vi "GeometricPatternMatch_Setting_UI.vi"(0 "Vision_Image In":T3(plugin-control), 1 "Coord?":bool, 3 "Type":string, 5 "List ROI Ref":refnum<vi>, 7 "AlgIn":T2, 9 "ProjectName":string="CDF", 11 "error in (no error)":errorcluster, 12 "ParameterIn":string, 14 "RootPath":path) -> (6 "ParameerOut":string, 10 "IMAQ Curve Parameters.ctlCancel?":bool, 15 "error out":errorcluster)   [LabVIEW 2019]
uses:
  Controls/V_Analysis_Type.ctl
  <vilib>/vision/Pattern Matching.llb/IMAQ Match Range Setting.ctl
  Controls/_UI Command Cluster/Pattern Match_UI Command.ctl
  <vilib>/Utility/miscctls.llb/LVPointTypeDef.ctl
  Controls/Analysis_Setting.ctl
  Controls/Geometric Match/Analysis_Geometric PatternMatch_Parameter.ctl
  <vilib>/vision/Image Controls.llb/IMAQ Image.ctl
  11e1650d-9a27-4c98-b785-94bb4e51b252.vi
  fe4c8c9f-3b30-4d10-b5c7-71603a67618a.vi
  c6f29bbc-09ff-4359-9596-1a03bc10ebeb.vi
  7765c890-54c4-40a3-a063-9b2138e01ba1.vi
  ff688e6c-f413-41b3-9d93-3794729c7324.vi
  <vilib>/JDP Science/JSONtext/JSON text to Variant.vi
  <vilib>/JDP Science/JSONtext/Variant to JSON Text.vi
  <vilib>/vision/NI_Vision_Development_Module.lvlib
  <vilib>/userdefined/High Color/IMAQdx.ctl
panel:
  out "ListROI":T1
  out "Algout":T2=enum."G_PatternMatching"
  in  "SetROI":bool
  out "ROI":T1
  out "Template Image":T3(plugin-control)
  in  "Cancel":bool
  in  "Done":bool
  in  "PatternMatchTab":T4(tab)
  in  "Show Curve":bool
  in  "Curve Extraction":T5={"Extraction Mode"=0, "Edge Threshold"=75, "Edge Filter Size"=1, "Min Length"=25, "Row Search Step Size"=15, "Column Search Step Size"=15, "Max Endpoint Gap"=10, "Closed"=FALSE, "Subpixel"=FALSE} {"Edge Filter Size" items=["Fine", "Normal", "Contour Tracing"]; "Edge Threshold" min=0 max=255 step=1; "Extraction Mode" items=["Normal", "Uniform Regions"]}
  in  "Y Position Offset":i32
  in  "X Position Offset":i32
  in  "Match Parameters":T6={"Number of Matches Requested"=1, "Minimum Match Score"=750.0, "Angle Ranges"=[]} {"Angle Ranges"."End Angle" min=-360 max=360; "Angle Ranges"."Start Angle" min=-360 max=360; "Minimum Match Score" min=0 max=1000; "Number of Matches Requested" min=1 max=9999}
  in  "Match Mode":T7={"Rotation"=TRUE, "Scale"=FALSE, "Occlusion"=FALSE, "Reserved"=FALSE, "Reserved"=FALSE, "Reserved"=FALSE}
  in  "Range Settings":T8[](array[typedef])=[{"Match Constraints"=0, "Min"=-180.0, "Max"=180.0}] {"Match Constraints" items=["Rotation Angle (degrees)", "Scale Factor (%)", "Occlusion (%)"]}
  out "Matches (pixel)":T9(array[cluster]) {"Correlation Score" format="%.2f"; "Curve Score" format="%.2f"; "Curve Score" format="%.2f"; "Occlusion %" format="%.2f"; "Bounding Box"."y" format="%.2f"; "Bounding Box"."x" format="%.2f"; "Position"."y" format="%.2f"; "Position"."x" format="%.2f"; "Score" format="%.2f"; "Scale" format="%.2f"; "Angle" format="%.2f"}
  in  "Vision_Image":T3(plugin-control)
  in  "Run Algorithm":bool
  in  "SetTemplate":bool
  # "Range"
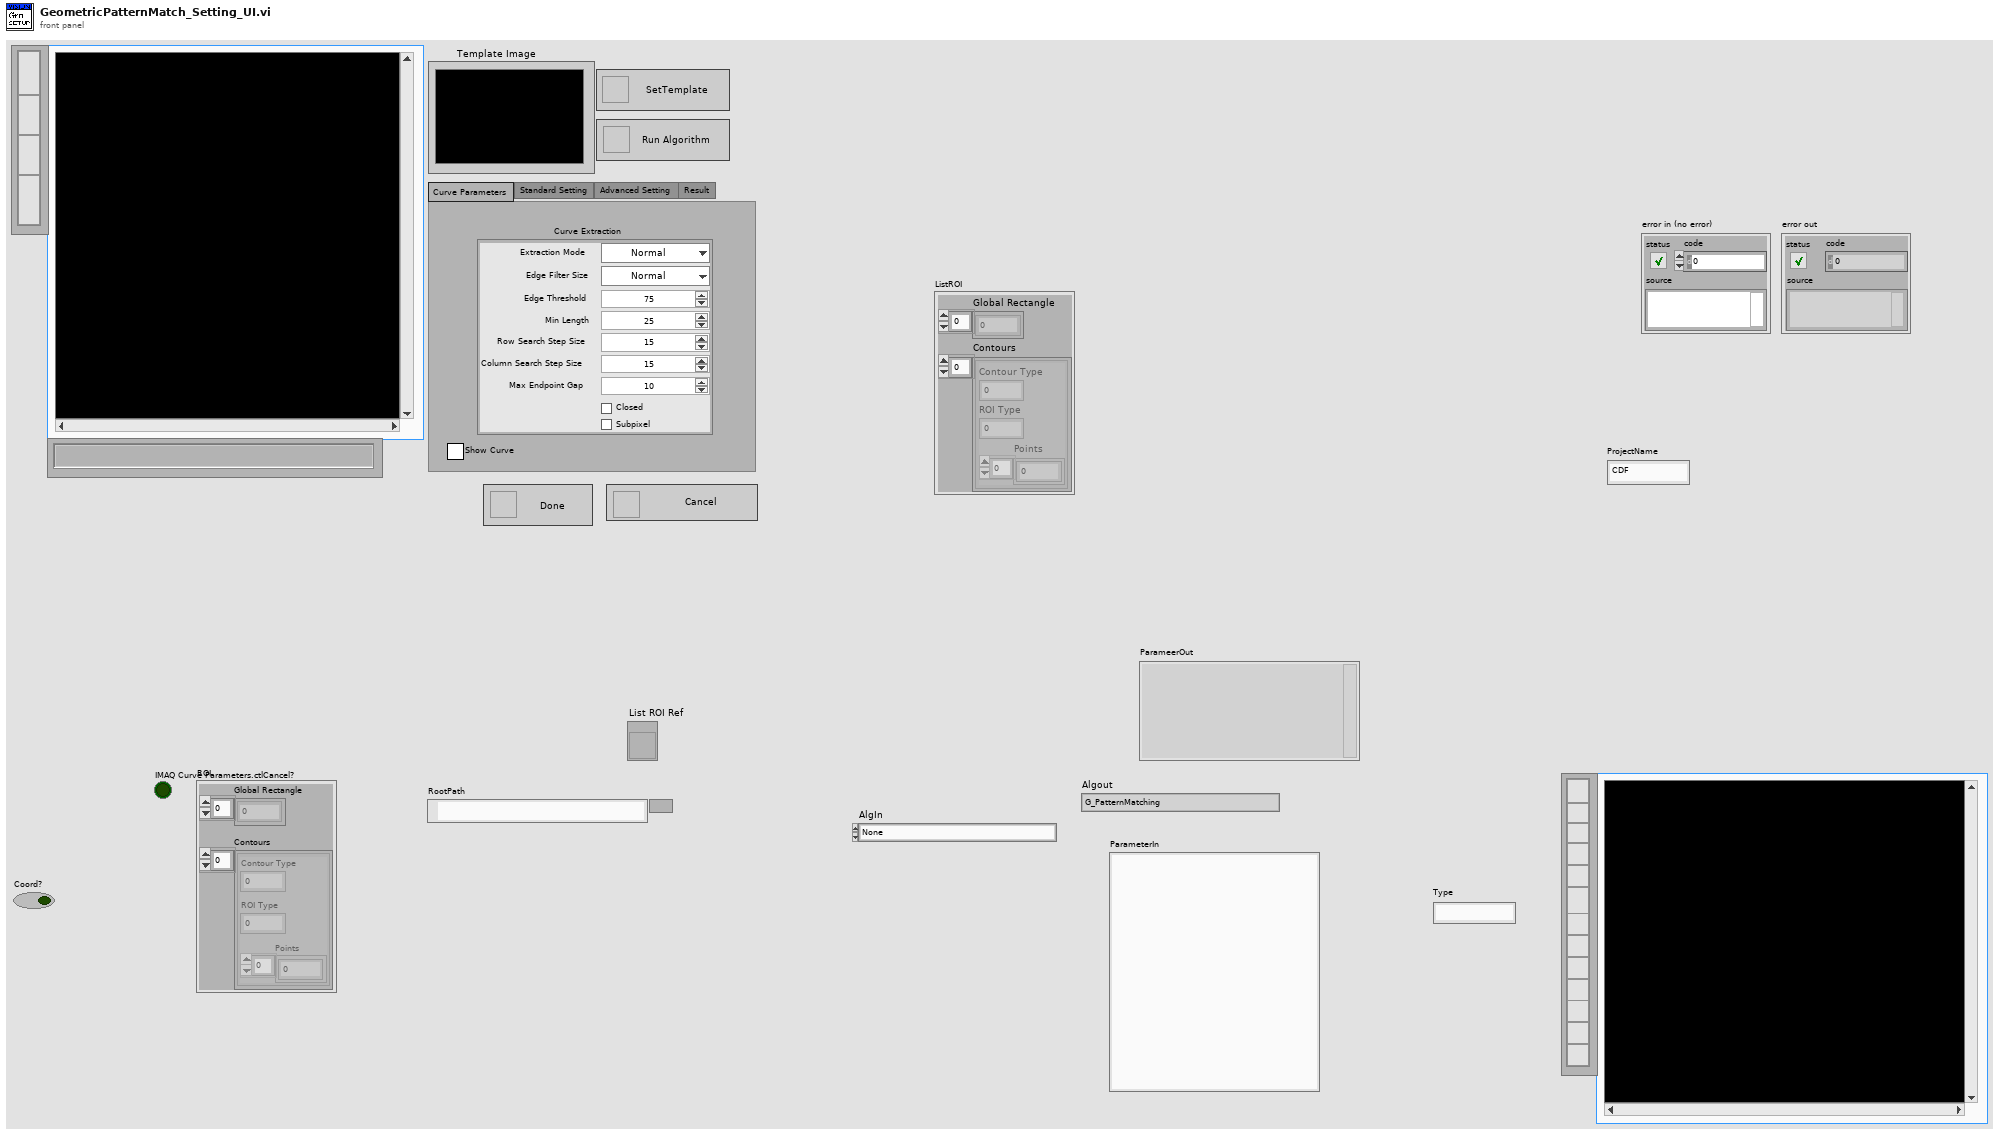
[diagram p1: front panel]
types:
  T1 = cluster{"Global Rectangle":i32[], "Contours":cluster{"Contour Type":u32, "ROI Type":u32, "Points":i32[]}[]}
  T2 = typedef "V_Analysis_Type.ctl" = enum16{"None", "C_Color Pattern Matching", "G_PatternMatching", "G_ShapeDectect", "G_GeometricMatch", "B_Area Check"}
  T3 = typedef "IMAQ Image.ctl" = refnum<image>
  T4 = enum32{"Curve Parameters", "Standard Setting", "Advanced Setting", "Result"}
  T5 = cluster{"Extraction Mode":u32, "Edge Threshold":i32, "Edge Filter Size":u32, "Min Length":i32, "Row Search Step Size":i32, "Column Search Step Size":i32, "Max Endpoint Gap":i32, "Closed":bool, "Subpixel":bool}
  T6 = cluster{"Number of Matches Requested":i32, "Minimum Match Score":sgl, "Angle Ranges":cluster{"Start Angle":sgl, "End Angle":sgl}[]}
  T7 = cluster{"Rotation":bool, "Scale":bool, "Occlusion":bool, "Reserved":bool, "Reserved":bool, "Reserved":bool}
  T8 = typedef "IMAQ Match Range Setting.ctl" = cluster{"Match Constraints":u32, "Min":dbl, "Max":dbl}
  T9 = cluster{"Position":cluster{"x":sgl, "y":sgl}, "Angle":sgl, "Scale":sgl, "Score":sgl, "Bounding Box":cluster{"x":sgl, "y":sgl}[], "Contrast Reversed":bool, "Occlusion %":sgl, "Curve Score":sgl, "Curve Score":sgl, "Correlation Score":sgl}[]
  T10 = typedef "Image Type" = u32
  T11 = typedef "Pattern Match_UI Command.ctl" = enum16{"Init", "Done", "Cancel", "RunAlgorithm", "SetTemplate", "SetROI", "ClearOverlay", "Load Template", "Draw Overlay", "Offset", "Draw Curve"}
  T12 = typedef "LVPointTypeDef.ctl" = cluster{"Horizontal":i16, "Vertical":i16}
  T13 = typedef "IMAQdx.ctl" = refnum<k21>
  T14 = typedef "Analysis_Geometric PatternMatch_Parameter.ctl" = cluster{"Curve Extraction":cluster{"Extraction Mode":u32, "Edge Threshold":i32, "Edge Filter Size":u32, "Min Length":i32, "Row Search Step Size":i32, "Column Search Step Size":i32, "Max Endpoint Gap":i32, "Closed":bool, "Subpixel":bool}, "X Position Offset":i32, "Y Position Offset":i32, "Match Parameters":cluster{"Number of Matches Requested":i32, "Minimum Match Score":sgl, "Angle Ranges":cluster{"Start Angle":sgl, "End Angle":sgl}[]}, "Template path":string, "Range Settings":T8[], "Match Mode":cluster{"Rotation":bool, "Scale":bool, "Occlusion":bool, "Reserved":bool, "Reserved":bool, "Reserved":bool}}
  T15 = typedef "Analysis_Setting.ctl" = cluster{"PreProcess":T2, "Parameter":string}
  T16 = enum8{"Enabled", "Disabled", "Disabled and Grayed Out"}
  T17 = typedef "ROI Descriptor" = cluster{"Global Rectangle":i32[], "Contours":cluster{"ID":enum32{"External", "Internal"}, "Type":u32, "Coordinates":i32[]}[]}
  T18 = cluster{"Position":cluster{"x":sgl, "y":sgl}, "Angle":sgl, "Scale":sgl, "Score":sgl, "Bounding Box":cluster{"x":sgl, "y":sgl}[]}[]
  T19 = typedef "IMAQ GM Match Report.ctl" = cluster{"Position":cluster{"x":sgl, "y":sgl}, "Angle":sgl, "Scale":sgl, "Score":sgl, "Bounding Box":cluster{"x":sgl, "y":sgl}[], "Contrast Reversed":bool, "Occlusion %":sgl, "Template Target Curve Score":sgl, "Target Template Curve Score":sgl, "Correlation Score":sgl}
  T20 = cluster{"Contour Type":u32, "ROI Type":u32, "Points":i32[]}[]
  T21 = cluster{"X Position Offset":i32, "Y Position Offset":i32}
  T22 = enum16{"Init", "Done", "Cancel", "RunAlgorithm", "SetTemplate", "SetROI", "ClearOverlay"}
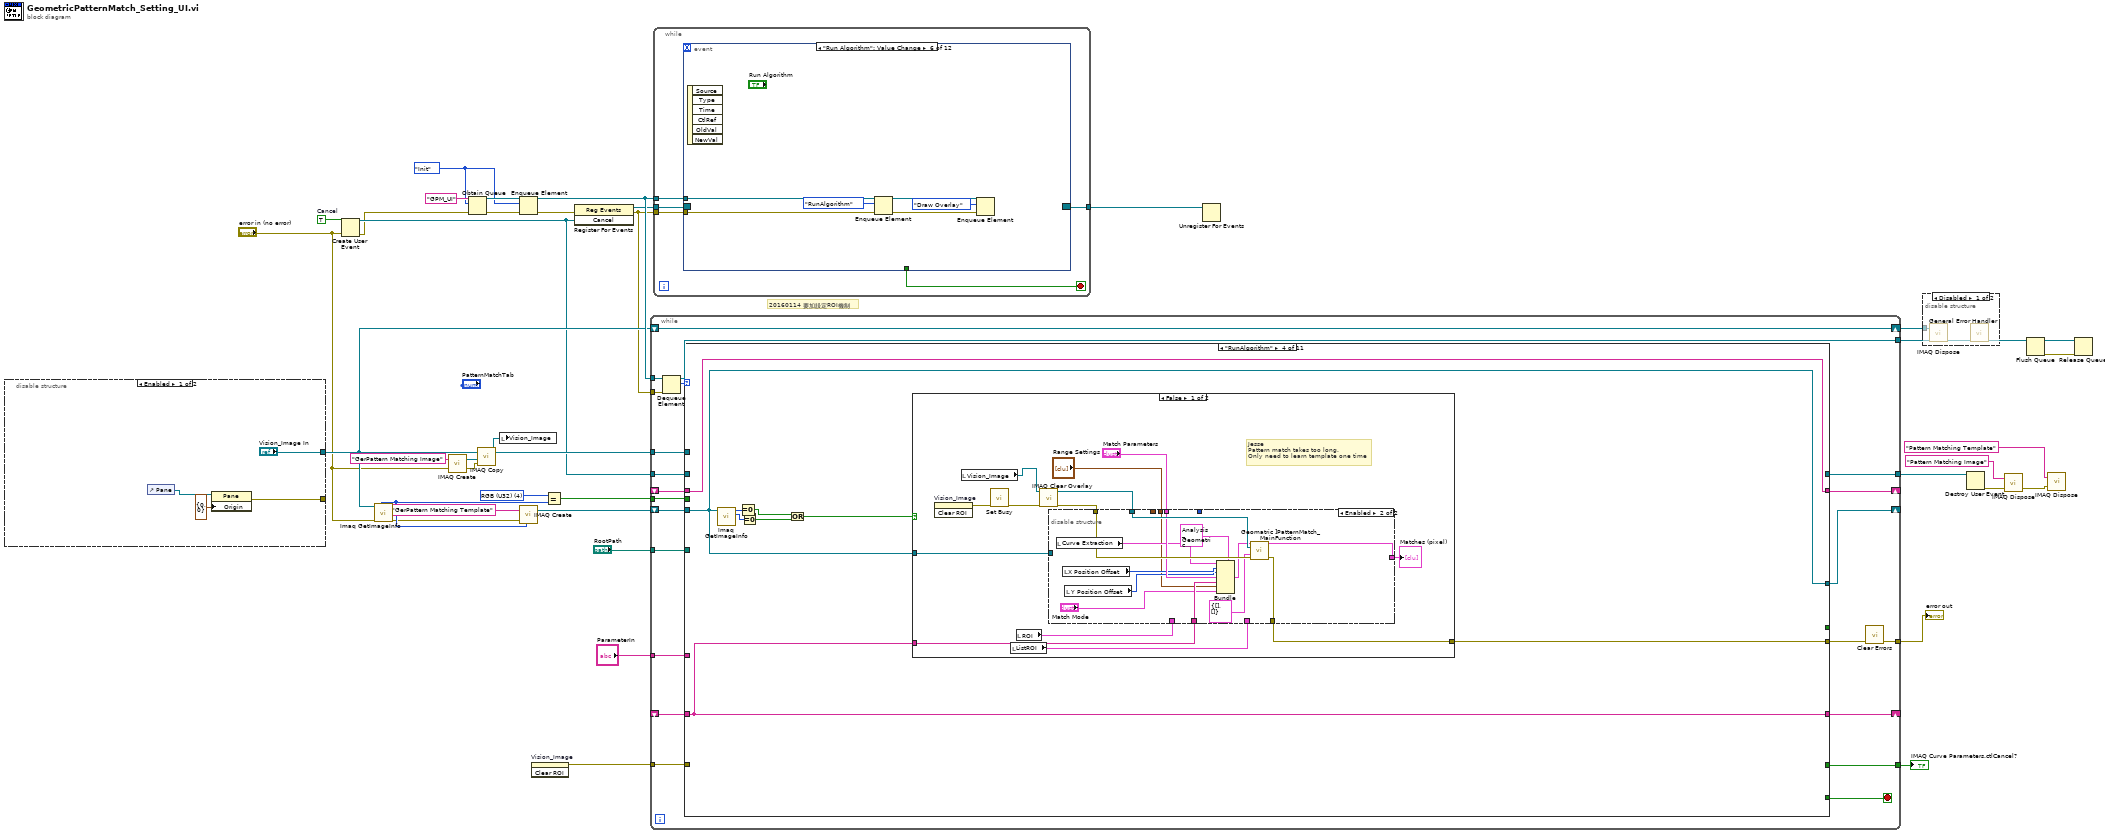
[diagram p0: block diagram]
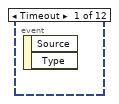
[diagram p2: hidden frame]
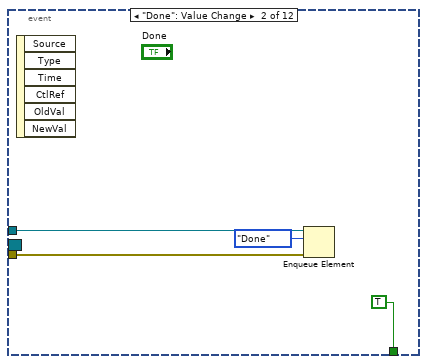
[diagram p3: hidden frame]
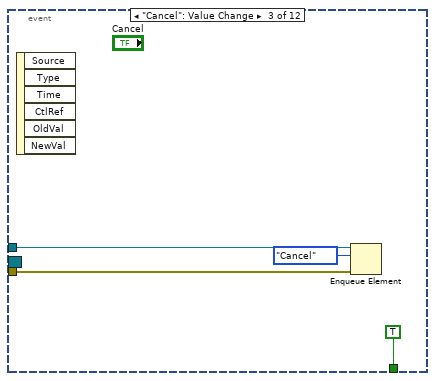
[diagram p4: hidden frame]
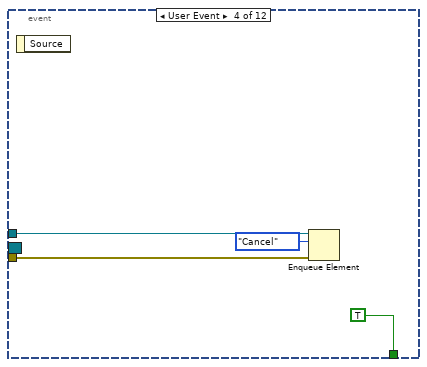
[diagram p5: hidden frame]
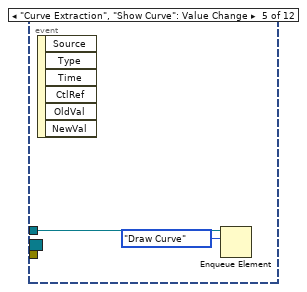
[diagram p6: hidden frame]
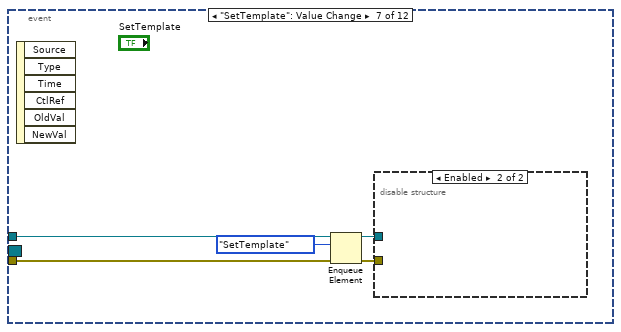
[diagram p7: hidden frame]
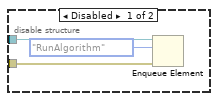
[diagram p8: hidden frame]
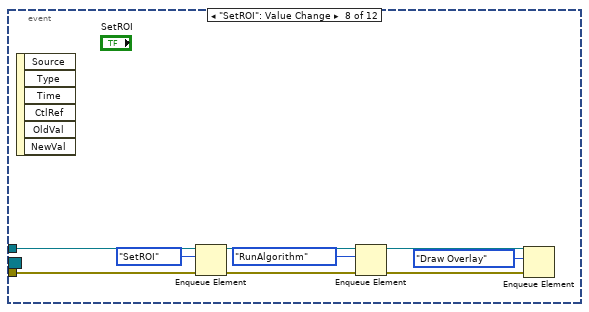
[diagram p9: hidden frame]
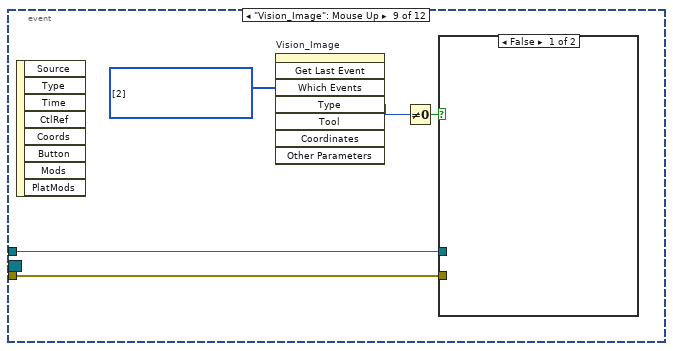
[diagram p10: hidden frame]
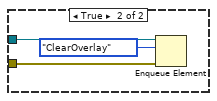
[diagram p11: hidden frame]
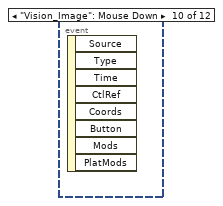
[diagram p12: hidden frame]
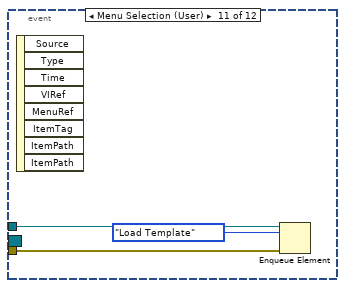
[diagram p13: hidden frame]
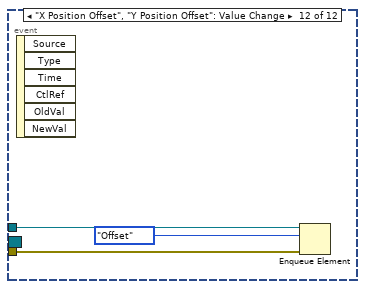
[diagram p14: hidden frame]
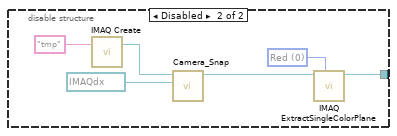
[diagram p15: hidden frame]
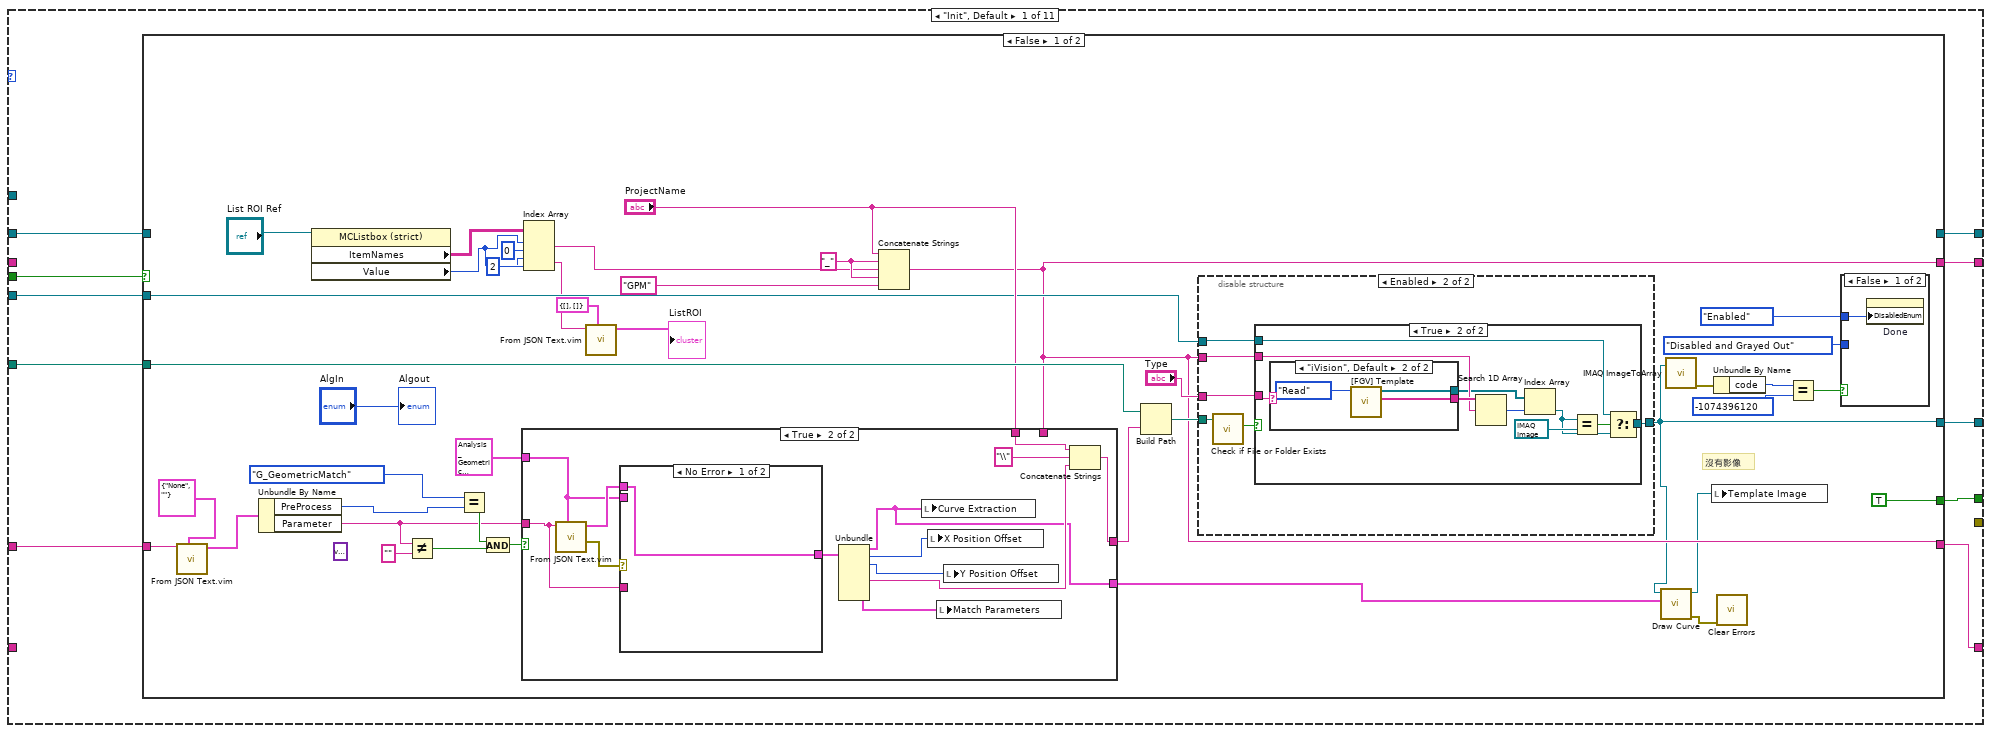
[diagram p17: hidden frame]
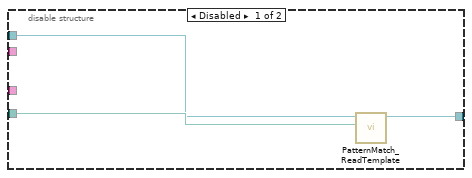
[diagram p18: hidden frame]
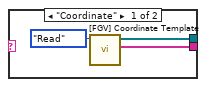
[diagram p20: hidden frame]
diagram:
  w18 = TRUE  # Cancel
  w20 = T10 4 items=["Grayscale (U8)", "Grayscale (I16)", "Grayscale (SGL)", "Complex (CSG)", "RGB (U32)", "HSL (U32)", "RGB (U64)", "Grayscale (U16)"] ("x")
  w19 = Pattern_Match_UI_Command."Init"
  # "20160114 要加設定ROI機制"
  n1 = disable-structure shown="Enabled" {
    disable-tunnel: ["Vision_Image In" w44] -> w24
    disable-tunnel: [w39 _] -> _
    frame Enabled {
      n2 = control-ref of="Pane"() -> (w41:refnum<vi>)
      n3 = property class="Pane"(reference=w41, "Origin"=T12 {"Horizontal"=0, "Vertical"=0}) -> (error out=w39:errorcluster)  [unwired: 1 in, 1 out]
    }
    frame Disabled {
      w43 = 0 items=["Red", "Green", "Blue", "Hue", "Saturation", "Luminance", "Value", "Intensity"] ("Color Plane")
      n4 = call "IMAQ Create"("Image Name"="tmp") -> ("New Image"=w46:T3)  [unwired: 4 in, 1 out]
      n5 = call "Camera_Snap.vi"("Camera Session In"=T13 "cam0", "Image In"=w46) -> ("New Image"=w45:T3)  [unwired: 8 in, 1 out]
      n6 = call "IMAQ ExtractSingleColorPlane"("Color Plane"=w43, "Image Src"=w45) -> ("Image Dst Out"=w44:T3)  [unwired: 2 in, 7 out]
    }
  }
  n7 = Create User Event(user event datatype=w18, error in="error in (no error)") -> (user event=w15:refnum<user-event>, error out=w6:errorcluster)
  n8 = call "Imaq GetImageInfo"("error in (no error)"="error in (no error)", "Image"=w24) -> ("error out"=w4:errorcluster, "Image Type"=w21:T10)  [unwired: 2 in, 6 out]
  n9 = call "IMAQ Create"("Image Name"="GerPattern Matching Image", "error in (no error)"="error in (no error)") -> ("New Image"=w33:T3, "error out"=w5:errorcluster)  [unwired: 3 in]
  n10 = Obtain Queue(name (unnamed)="GPM_UI", element data type=w19, error in (no error)=w6) -> (queue out=w30:refnum<queue>, error out=w29:errorcluster)  [unwired: 2 in, 1 out]
  n11 = call "IMAQ Copy"("error in (no error)"=w5, "Image Dst"=w33, "Image Src"=w24) -> ("Image Dst Out"=w32:T3)  [unwired: 3 in, 1 out]
  n12 = local write "Vision_Image"(w32) -> ()
  n13 = Enqueue Element(queue=w30, element=w19, error in (no error)=w29) -> (queue out=w26:refnum<queue>, error out=w12:errorcluster)  [unwired: 1 in, 1 out]
  n14 = call "IMAQ Create"("Image Name"="GerPattern Matching Template", "Image Type"=w21, "error in (no error)"=w4) -> ("New Image"=w23:T3)  [unwired: 2 in, 1 out]
  n15 = invoke on="Vision_Image" class="ImageControl" method="Clear ROI"() -> (error out=w35:errorcluster)  [unwired: 3 in, 2 out]
  n16 = Equal?(x=w20, y=w21) -> (x = y?=w16:bool)
  n17 = register-events(error in=w12, w15) -> (reference out=w17:refnum<event-registration>, error out=w11:errorcluster)  [unwired: 1 in]
  n18 = while {
    shift-right: [w70] -> w38
    shift-left: w24 -> [w70]
    tunnel: [w66] -> w37
    tunnel: w35 -> [w52]
    tunnel: w32 -> [w69]
    tunnel: w26 -> [w64]
    tunnel: w11 -> [w62]
    tunnel: [w61] -> w25
    shift-right: [w60] -> _
    shift-left: _ -> [w59]
    shift-right: [w57] -> _
    shift-left: w23 -> [w68]
    shift-right: [w58] -> _
    shift-left: _ -> [w67]
    tunnel: "RootPath" -> [w56]
    tunnel: w16 -> [w55]
    tunnel: w15 -> [w54]
    tunnel: [w53] -> w14
    tunnel: [w51] -> w2
    tunnel: "ParameterIn" -> [w49]
    stop <- w65 stop-if-true
    n19 = Dequeue Element(queue=w64, error in (no error)=w62) -> (queue out=w61:refnum<queue>, element=w63:T11)  [unwired: 1 in, 2 out]
    n20 = case shown="\"RunAlgorithm\"" w63 {
      tunnel: [_ TRUE w205 _ _ _ _ _ _ _ _] -> w65
      tunnel: w69 -> [_ w194 w204 _ w262 _ _ _ _ _ w447]
      tunnel: w68 -> [w75 _ w203 w209 w264 w311 w380 w390 w404 w419 w445]
      tunnel: [_ _ w205 _ _ _ _ _ _ _ _] -> w66
      tunnel: w67 -> [_ w183 w201 w207 w263 w312 w381 w391 w405 w424 w444]
      tunnel: [w79 w193 w202 w214 w265 w313 w382 w392 w406 _ w446] -> w60
      tunnel: w59 -> [_ w193 w202 w214 w265 w313 w382 w392 w406 _ w446]
      tunnel: [w77 w183 w201 w207 w263 w312 w381 w391 w405 w424 w444] -> w58
      tunnel: [w80 T3 refnum ("Template Out") T3 refnum ("Template Out") w209 w264 w308 w380 w390 w396 w426 w445] -> w57
      tunnel: [w78 FALSE _ _ _ w310 _ _ _ _ _] -> _
      tunnel: w56 -> [w76 _ _ _ _ w309 _ _ w403 w425 _]
      tunnel: w55 -> [w74 _ _ _ _ _ _ _ _ _ _]
      tunnel: w54 -> [w73 w190 w199 _ _ _ _ _ _ _ _]
      tunnel: [w72 w190 w199 _ _ _ _ _ _ _ _] -> w53
      tunnel: w52 -> [_ _ _ _ w259 _ _ _ _ _ _]
      tunnel: [_ _ _ w206 _ _ _ _ _ _ _] -> w50
      tunnel: w49 -> [w71 _ _ _ _ _ _ _ _ _ _]
      frame "Init", Default {
        n21 = case shown="False" w74 {
          tunnel: [w83 _] -> w80
          tunnel: [w87 _] -> w79
          tunnel: [TRUE _] -> w78
          tunnel: [w87 _] -> w77
          tunnel: w76 -> [w120 _]
          tunnel: w75 -> [w110 _]
          tunnel: w73 -> [_ w176]
          tunnel: [_ w174] -> w72
          tunnel: w71 -> [w89 _]
          frame False {
            (unwired) variant
            w117 = "_" ("string")
            # "沒有影像"
            n22 = call "From JSON Text.vim"("Data Type and Default Value"=T15 {"PreProcess"=enum."None", "Parameter"=""} ("Analysis_Setting In"), "JSON"=w89) -> ("Data out"=w90:T15)  [unwired: 8 in, 1 out]
            n23 = Unbundle By Name(w90) -> ("PreProcess"=w88:T2, "Parameter"=w112:string)
            n24 = property class="MCListbox (strict)"(reference="List ROI Ref") -> ("ItemNames"=w97:string[][], "Value"=w96:i32)  [unwired: 1 in, 2 out]
            n25 = Not Equal?(x=w112, y="") -> (x != y?=w115:bool)
            n26 = Equal?(x=V_Analysis_Type."G_GeometricMatch", y=w88) -> (x = y?=w116:bool)
            n27 = And(x=w116, y=w115) -> (x .and. y?=w113:bool)
            n28 = Index Array(array=w97, index (row) #1=w96, index (col) #1=0 ("disabled index (col)"), index (row) #2=w96, index (col) #2=2 ("disabled index (col)")) -> (element #1=w95:string, element #2=w93:string)
            n29 = call "From JSON Text.vim"("Data Type and Default Value"=T1 {"Global Rectangle"=[], "Contours"=[]} ("ROI"), "JSON"=w93) -> ("Data out"=→"ListROI":T1)  [unwired: 8 in, 1 out]
            n30 = Concatenate Strings("ProjectName", w117, w95, w117, "GPM" ("string")) -> (w87:string)
            n31 = case shown="True" w113 {
              tunnel: [w152 w166] -> w86
              tunnel: "ProjectName" -> [w153 w168]
              tunnel: w112 -> [_ w170]
              tunnel: w87 -> [w154 _]
              tunnel: T14 {"Curve Extraction"={"Extraction Mode"=0, "Edge Threshold"=75, "Edge Filter Size"=1, "Min Length"=25, "Row Search Step Size"=15, "Column Search Step Size"=15, "Max Endpoint Gap"=10, "Closed"=FALSE, "Subpixel"=FALSE}, "X Position Offset"=0, "Y Position Offset"=0, "Match Parameters"={"Number of Matches Requested"=1, "Minimum Match Score"=750.0, "Angle Ranges"=[]}, "Template path"="", "Range Settings"=[], "Match Mode"={"Rotation"=TRUE, "Scale"=FALSE, "Occlusion"=FALSE, "Reserved"=FALSE, "Reserved"=FALSE, "Reserved"=FALSE}} ("Cluster") -> [w151 w165]
              tunnel: [w150 w159] -> w82
              frame False {
                n32 = invoke on="Y Position Offset" class="DigNum (strict)" method="Reinit To Default"() -> ()  [unwired: 3 in, 3 out]
                n33 = invoke on="X Position Offset" class="DigNum (strict)" method="Reinit To Default"() -> ()  [unwired: 3 in, 3 out]
                n34 = Unbundle By Name(w151) -> ("Curve Extraction"=w150:T5)
                n35 = case shown="True" "Coord?" {
                  frame False {
                    n36 = invoke on="Match Parameters" class="Clust (strict)" method="Reinit To Default"() -> ()  [unwired: 3 in, 3 out]
                  }
                  frame True {
                    n37 = local write "Match Parameters"(T6 {"Number of Matches Requested"=1, "Minimum Match Score"=750.0, "Angle Ranges"=[{"Start Angle"=0.0, "End Angle"=360.0}]} ("Match Parameters")) -> ()
                  }
                }
                n38 = Concatenate Strings(w153, "\\" ("string"), w154) -> (w152:string)
                "ROI" <- T1 {"Global Rectangle"=[], "Contours"=[]} ("ROI")
              }
              frame True {
                n39 = call "From JSON Text.vim"("Data Type and Default Value"=w165, "JSON"=w170) -> ("error out"=w171:errorcluster, "Data out"=w169:T14)  [unwired: 8 in]
                n40 = case shown="No Error" w171 {
                  tunnel: w170 -> [_ _]
                  tunnel: [w172 w173] -> w164
                  tunnel: w169 -> [w172 _]
                  tunnel: w165 -> [_ w173]
                  frame No Error {
                  }
                  frame Error {
                  }
                }
                n41 = Unbundle(w164) -> ("Curve Extraction"=w159:T5, "X Position Offset"=w163:i32, "Y Position Offset"=w162:i32, "Match Parameters"=w161:T6, "Template path"=w160:string)  [unwired: 2 out]
                n42 = local write "Curve Extraction"(w159) -> ()
                n43 = local write "X Position Offset"(w163) -> ()
                n44 = local write "Match Parameters"(w161) -> ()
                n45 = local write "Y Position Offset"(w162) -> ()
                n46 = Concatenate Strings(w168, "\\" ("string"), w160) -> (w166:string)
              }
            }
            n47 = Build Path(base path=w120, name or relative path=w86) -> (appended path=w111:path)
            n48 = disable-structure shown="Enabled" {
              disable-tunnel: w111 -> [w124 w129]
              disable-tunnel: w110 -> [w123 w126]
              disable-tunnel: [w122 w127] -> w83
              disable-tunnel: w87 -> [_ w130]
              disable-tunnel: "Type" -> [_ w125]
              frame Disabled {
                n49 = call "PatternMatch_ReadTemplate.vi"("template path"=w124, "Template"=w123) -> ("Template Out"=w122:T3)  [unwired: 8 in, 1 out]
              }
              frame Enabled {
                n50 = call <vilib>:"Check if File or Folder Exists.vi"("path"=w129) -> ("file or folder exists?"=w128:bool)  [unwired: 8 in, 2 out]
                n51 = case shown="True" w128 {
                  tunnel: w130 -> [_ w140]
                  tunnel: [w131 w132] -> w127
                  tunnel: w126 -> [w131 w134]
                  tunnel: w125 -> [_ w137]
                  frame False {
                  }
                  frame True {
                    n52 = case shown="\"iVision\", Default" w137 {
                      tunnel: [w143 w146] -> w141
                      tunnel: [w144 w145] -> w138
                      frame "Coordinate" {
                        n53 = call "[FGV] Coordinate Template.vi"("Command"=enum16{"Initialize", "Save", "Read"}."Read") -> ("Image Name Array"=w143:string[], "Image Array"=w144:T3[])  [unwired: 8 in, 1 out]
                      }
                      frame "iVision", Default {
                        n54 = call "[FGV] Template.vi"("Command"=enum16{"Initialize", "Save", "Read"}."Read") -> ("Image Name Array"=w146:string[], "Image Array"=w145:T3[])  [unwired: 8 in, 1 out]
                      }
                    }
                    n55 = Search 1D Array(1D array=w141, element=w140) -> (index of element=w139:i32)  [unwired: 1 in]
                    n56 = Index Array(array=w138, index=w139) -> (element=w133:T3)
                    n57 = Equal?(x=w133, y=T3 refnum) -> (x = y?=w135:bool)
                    n58 = Select(t=w134, s=w135, f=w133) -> (s? t:f=w132:T3)
                  }
                }
              }
            }
            n59 = call "Draw Curve.vi"("Curve Extraction"=w82, "Refnum in"=w83) -> ("error out"=w81:errorcluster, "Refnum out"=w84:T3)  [unwired: 8 in]
            n60 = call "IMAQ ImageToArray"("Image"=w83) -> ("error out"=w107:errorcluster)  [unwired: 3 in, 4 out]
            n61 = local write "Template Image"(w84) -> ()
            n62 = Unbundle By Name(w107) -> ("code"=w106:i32)
            n63 = call <vilib>:"Clear Errors.vi"("error in (no error)"=w81) -> ()  [unwired: 5 in, 2 out]
            n64 = Equal?(x=w106, y=-1074396120) -> (x = y?=w104:bool)
            n65 = case shown="False" w104 {
              tunnel: T16."Disabled and Grayed Out" ("Disabled") -> [_ w149]
              tunnel: T16."Enabled" ("Disabled") -> [w148 _]
              frame False {
                n66 = property on="Done" class="Bool"("DisabledEnum"=w148) -> ()  [unwired: 2 in, 2 out]
              }
              frame True {
                n67 = property on="Done" class="Bool"("DisabledEnum"=w149) -> ()  [unwired: 2 in, 2 out]
              }
            }
            "Algout" <- "AlgIn"
          }
          frame True {
            # "輸入進來若是RGB則關閉"
            n68 = One Button Dialog(message="The Input Image Error,Image RGB", button name ("OK")="Cancel") -> (true=w175:bool)
            n69 = Generate User Event(user event=w176, event data cluster=w175) -> (user event out=w174:refnum<user-event>)  [unwired: 2 in, 1 out]
          }
        }
      }
      frame "Done" {
        w196 = T15 {"PreProcess"=enum."None", "Parameter"=""}  # Analysis_Setting
        n70 = call "IMAQ Dispose"("Image"=w194) -> ()  [unwired: 5 in, 1 out]
        n71 = local read "Y Position Offset"() -> (w181:i32)
        n72 = local read "X Position Offset"() -> (w182:i32)
        n73 = local read "Curve Extraction"() -> (w184:T5)
        n74 = local read "Match Parameters"() -> (w195:T6)
        n75 = local read "Range Settings"() -> (w180:T8[])
        n76 = local read "Match Mode"() -> (w179:T7)
        n77 = Bundle By Name(cluster=T14 {"Curve Extraction"={"Extraction Mode"=0, "Edge Threshold"=75, "Edge Filter Size"=1, "Min Length"=25, "Row Search Step Size"=15, "Column Search Step Size"=15, "Max Endpoint Gap"=10, "Closed"=FALSE, "Subpixel"=FALSE}, "X Position Offset"=0, "Y Position Offset"=0, "Match Parameters"={"Number of Matches Requested"=1, "Minimum Match Score"=750.0, "Angle Ranges"=[]}, "Template path"="", "Range Settings"=[], "Match Mode"={"Rotation"=TRUE, "Scale"=FALSE, "Occlusion"=FALSE, "Reserved"=FALSE, "Reserved"=FALSE, "Reserved"=FALSE}} ("Cluster"), "Curve Extraction"=w184, "Match Parameters"=w195, "X Position Offset"=w182, "Y Position Offset"=w181, "Template path"=w183, "Range Settings"=w180, "Match Mode"=w179) -> (w189:T14)
        n78 = call "To JSON Text.vim"("Anything"=w189) -> ("<JSON>"=w188:string)  [unwired: 9 in, 1 out]
        n79 = Bundle By Name(cluster=w196, "PreProcess"=V_Analysis_Type."G_GeometricMatch" ("Analysis"), "Parameter"=w188) -> (w187:T15)
        n80 = call "To JSON Text.vim"("Anything"=w187) -> ("<JSON>"=→"ParameerOut":string)  [unwired: 9 in, 1 out]
      }
      frame "Cancel" {
        w205 = TRUE
        n81 = call "IMAQ Dispose"("Image"=w203) -> ()  [unwired: 5 in, 1 out]
        n82 = call "IMAQ Dispose"("Image"=w204) -> ()  [unwired: 5 in, 1 out]
      }
      frame "RunAlgorithm" {
        n83 = call "Imaq GetImageInfo"("Image"=w209) -> ("Y Resolution"=w213:i32, "X Resolution"=w212:i32)  [unwired: 3 in, 6 out]
        n84 = Equal To 0?(x=w212) -> (x = 0?=w211:bool)
        n85 = Equal To 0?(x=w213) -> (x = 0?=w210:bool)
        n86 = Or(x=w211, y=w210) -> (x .or. y?=w208:bool)
        n87 = case shown="False" w208 {
          tunnel: w209 -> [w221 _]
          tunnel: w207 -> [w220 _]
          tunnel: [w219 _] -> w206
          frame False {
            # "Jesse\nPattern match takes too long.\nOnly need to learn template one time"
            n88 = invoke on="Vision_Image" class="ImageControl" method="Clear ROI"() -> (error out=w227:errorcluster)  [unwired: 3 in, 2 out]
            n89 = local read "Vision_Image"() -> (w215:T3)
            n90 = call <vilib>:"Set Busy.vi"("error in (no error)"=w227) -> ("error out"=w226:errorcluster)  [unwired: 9 in, 1 out]
            n91 = local read "ListROI"() -> (w218:T1)
            n92 = local read "ROI"() -> (w222:T1)
            n93 = call "IMAQ Clear Overlay"("error in (no error)"=w226, "Image"=w215) -> ("error out"=w223:errorcluster, "Image Out"=w225:T3)  [unwired: 8 in]
            n94 = disable-structure shown="Enabled" {
              disable-tunnel: w221 -> [w237 _]
              disable-tunnel: w223 -> [w236 w251]
              disable-tunnel: "Match Parameters" -> [w234 w247]
              disable-tunnel: _ -> [w233 _]
              disable-tunnel: _ -> [w232 _]
              disable-tunnel: w225 -> [w231 w252]
              disable-tunnel: [w230 w253] -> w217
              disable-tunnel: w222 -> [w228 _]
              disable-tunnel: w220 -> [_ w250]
              disable-tunnel: [_ w249] -> w219
              disable-tunnel: w218 -> [_ _]
              disable-tunnel: "Range Settings" -> [_ w242]
              frame Disabled {
                w239 = 0 items=["All", "Low Discrepancy Sampling", "Grayscale Value Pyramid", "Gradients Pyramid"] ("Algorithm")
                n95 = call "IMAQ Learn Pattern 4"("Algorithm"=w239, "error in (no error)"=w236, "Angle Range"=cluster{"Start Angle":sgl, "End Angle":sgl} {"Start Angle"=0.0, "End Angle"=360.0}, "Image"=w237) -> ("error out"=w235:errorcluster, "Template Image Out"=w229:T3)  [unwired: 5 in, 1 out]
                n96 = call "IMAQ Match Pattern 4"("Image"=w231, "Algorithm"=w233, "Template Image"=w229, "ROI Descriptor"=w228, "Parameters"=w234, "error in (no error)"=w235, "Advanced Options"=w232) -> ("Matches (pixel)"=w230:T18)  [unwired: 4 in, 4 out]
              }
              frame Enabled {
                n97 = local read "Curve Extraction"() -> (w246:T5)
                n98 = local read "X Position Offset"() -> (w245:i32)
                n99 = local read "Y Position Offset"() -> (w244:i32)
                n100 = Bundle(cluster=T14 {"Curve Extraction"={"Extraction Mode"=0, "Edge Threshold"=75, "Edge Filter Size"=1, "Min Length"=25, "Row Search Step Size"=15, "Column Search Step Size"=15, "Max Endpoint Gap"=10, "Closed"=FALSE, "Subpixel"=FALSE}, "X Position Offset"=0, "Y Position Offset"=0, "Match Parameters"={"Number of Matches Requested"=1, "Minimum Match Score"=750.0, "Angle Ranges"=[]}, "Template path"="", "Range Settings"=[], "Match Mode"={"Rotation"=TRUE, "Scale"=FALSE, "Occlusion"=FALSE, "Reserved"=FALSE, "Reserved"=FALSE, "Reserved"=FALSE}} ("Cluster"), "Curve Extraction"=w246, "X Position Offset"=w245, "Y Position Offset"=w244, "Match Parameters"=w247, "Template path"=w250, "Range Settings"=w242, "Match Mode"="Match Mode") -> (w243:T14)
                n101 = call "Geomatric ]PatternMatch_MainFunction.vi"("Geomatric Match Parameter"=w243, "Vision_Image In"=w252, "ROI Descriptor"=T17 {"Global Rectangle"=[], "Contours"=[]}, "error in"=w251) -> ("Matches (pixel)"=w253:T19[], "error out"=w249:errorcluster)  [unwired: 7 in, 3 out]
              }
            }
            "Matches (pixel)" <- w217
          }
          frame True {
            n102 = One Button Dialog(message="No Template is Set~!!!\nPlease Set Template Before Analyze~!!") -> ()  [unwired: 1 in, 1 out]
          }
        }
      }
      frame "Draw Overlay" {
        n103 = call "IMAQ Clear Overlay"("error in (no error)"=w259, "Image"=w262) -> ("error out"=w260:errorcluster, "Image Out"=w261:T3)  [unwired: 8 in]
        n104 = local read "Matches (pixel)"() -> (w255:T9)
        n105 = for {
          tunnel: w255 -> [w285] mode=indexing
          tunnel: w260 -> [w281]
          shift-right: [w279] -> w266
          shift-left: w261 -> [w284]
          tunnel: [w278] -> w257
          w280 = u32 16711680 ("Color")
          n106 = Unbundle By Name(w285) -> ("Position"=w283:cluster{"x":sgl, "y":sgl}, "Bounding Box"=w282:cluster{"x":sgl, "y":sgl}[])
          n107 = To Long Integer(number=w283) -> (32bit integer=w277:cluster{"x":i32, "y":i32})
          n108 = To Long Integer(number=w282) -> (32bit integer=w286:cluster{"x":i32, "y":i32}[])
          n109 = Unbundle(w277) -> ("x"=w275:i32, "y"=w274:i32)
          n110 = Bundle(cluster=w277, "x"=w275, "y"=w274) -> (w276:cluster{"x":i32, "y":i32})
          n111 = Bundle("x"=w275, "y"=w274, "x"=w275, "y"=w274) -> (w301:cluster{"x":i32, "y":i32, "x":i32, "y":i32})  [unwired: 1 out]
          n112 = Add(x=w301, y=cluster{"y":i32, "x":i32, "y":i32, "x":i32} {"y"=-5, "x"=-5, "y"=6, "x"=6}) -> (x+y=w299:cluster{i32, i32, i32, i32})
          n113 = call "IMAQ Overlay Oval"("Color"=w280, "error in (no error)"=w281, "Bounding Rectangle"=w299, "Image"=w284) -> ("error out"=w289:errorcluster, "Image Out"=w303:T3)  [unwired: 2 in, 4 out]
          n114 = Subtract(x=w276, y=cluster{"x":i32, "y":i32} {"x"=10, "y"=0}) -> (x-y=w297:cluster{"x":i32, "y":i32})
          n115 = Add(x=w297, y=cluster{"x":i32, "y":i32} {"x"=20, "y"=0}) -> (x+y=w295:cluster{"x":i32, "y":i32})
          n116 = call "IMAQ Overlay Line"("Color"=w280, "error in (no error)"=w289, "End Point"=w295, "Start Point"=w297, "Image"=w303) -> ("error out"=w288:errorcluster, "Image Out"=w290:T3)  [unwired: 1 in, 4 out]
          n117 = Subtract(x=w276, y=cluster{"x":i32, "y":i32} {"x"=0, "y"=10}) -> (x-y=w293:cluster{"x":i32, "y":i32})
          n118 = Add(x=w293, y=cluster{"x":i32, "y":i32} {"x"=0, "y"=20}) -> (x+y=w294:cluster{"x":i32, "y":i32})
          n119 = call "IMAQ Overlay Line"("Color"=w280, "error in (no error)"=w288, "End Point"=w294, "Start Point"=w293, "Image"=w290) -> ("error out"=w287:errorcluster, "Image Out"=w302:T3)  [unwired: 1 in, 4 out]
          n120 = call "IMAQ Overlay Multiple Lines"("Color"=w280, "error in (no error)"=w287, "Line End Points"=w286, "Image"=w302) -> ("error out"=w278:errorcluster, "Image Out"=w279:T3)  [unwired: 2 in, 4 out]
        }
        n121 = disable-structure shown="Enabled" {
          disable-tunnel: w266 -> [w271 w273]
          disable-tunnel: [w270 w273] -> w258
          disable-tunnel: w257 -> [w269 w272]
          disable-tunnel: [w268 w272] -> w256
          frame Disabled {
            n122 = local read "ListROI"() -> (w267:T1)
            n123 = call "IMAQ Overlay ROI"("error in (no error)"=w269, "ROI Descriptor"=w267, "Image"=w271) -> ("error out"=w268:errorcluster, "Image Out"=w270:T3)  [unwired: 7 in]
          }
          frame Enabled {
          }
        }
        n124 = call <vilib>:"Unset Busy.vi"("error in (no error)"=w256) -> ()  [unwired: 10 in, 1 out]
        n125 = local write "Vision_Image"(w258) -> ()
      }
      frame "SetTemplate" {
        # "沒有影像"
        # "-1074396120"
        n126 = call "Imaq GetImageInfo"("Image"=w311) -> ("error out"=w307:errorcluster)  [unwired: 3 in, 7 out]
        n127 = Unbundle By Name(w307) -> ("code"=w306:i32)
        n128 = Equal?(x=w306, y=-1074396120) -> (x = y?=w304:bool)
        n129 = case shown="False" w304 {
          tunnel: [w316 TRUE] -> w314
          frame False {
            n130 = Two Button Dialog(message="Template Already Exist, You Sure to Create New Template?") -> (T button?=w316:bool)  [unwired: 2 in]
          }
          frame True {
          }
        }
        n131 = case shown="True" w314 {
          tunnel: w311 -> [w318 w324]
          tunnel: w312 -> [_ w323]
          tunnel: [_ w322] -> w310
          tunnel: w309 -> [_ w321]
          tunnel: [w318 w320] -> w308
          frame False {
          }
          frame True {
            n132 = property on="Vision_Image" class="ImageControl"() -> ("ROI"=w328:T1)  [unwired: 2 in, 2 out]
            n133 = Unbundle By Name(w328) -> ("Contours"=w327:T20, "Global Rectangle"=w319:i32[])
            n134 = Array Size(array=w327) -> (size(s)=w326:i32)
            n135 = Not Equal To 0?(x=w326) -> (x != 0?=w325:bool)
            n136 = case shown="True" w325 {
              tunnel: w319 -> [_ w365]
              tunnel: w324 -> [w329 w364]
              tunnel: w323 -> [_ w348]
              tunnel: [_ TRUE] -> w322
              tunnel: w321 -> [_ w344]
              tunnel: [w329 w331] -> w320
              frame False {
                n137 = One Button Dialog(message="Please Select Template On the Image") -> ()  [unwired: 1 in, 1 out]
              }
              frame True {
                n138 = local read "ProjectName"() -> (w343:string)
                n139 = local read "X Position Offset"() -> (w341:i32)
                n140 = local read "Y Position Offset"() -> (w340:i32)
                n141 = call <vilib>:"Set Busy.vi"() -> ("error out"=w356:errorcluster)  [unwired: 10 in, 1 out]
                n142 = local read "Curve Extraction"() -> (w338:T5)
                n143 = Build Path(base path=w344, name or relative path=w343) -> (appended path=w345:path)
                n144 = Bundle("X Position Offset"=w341, "Y Position Offset"=w340) -> (w342:T21)  [unwired: 1 in]
                n145 = call "[FGV] Template.vi"("Command"=enum16{"Initialize", "Save", "Read"}."Read") -> ("Image Name Array"=w349:string[])  [unwired: 8 in, 2 out]
                n146 = call "IMAQ Extract"("Optional Rectangle"=w365, "error in (no error)"=w356, "Image Dst"=w364, "Image Src"="Vision_Image") -> ("error out"=w337:errorcluster, "Image Dst Out"=w357:T3)  [unwired: 6 in]
                n147 = Build Path(base path=w345, name or relative path=w348) -> (appended path=w361:path)
                n148 = Search 1D Array(1D array=w349, element=w348) -> (index of element=w350:i32)  [unwired: 1 in]
                n149 = call "IMAQ Setup Learn Geometric Pattern 2"("error in (no error)"=w337, "Curve Parameters"=w338) -> ("error out"=w336:errorcluster, "Learn Geometric Pattern 2 Setup Data"=w339:string)
                n150 = Less Than 0?(x=w350) -> (x < 0?=w347:bool)
                n151 = call "IMAQ Learn Geometric Pattern 3"("Template Image"=w357, "Origin Offset"=w342, "Learn Geometric Pattern 2 Setup Data"=w339, "error in (no error)"=w336) -> ("Template Image Out"=w346:T3, "error out"=w355:errorcluster)  [unwired: 10 in]
                n152 = case shown="True" w347 {
                  tunnel: w349 -> [_ w368]
                  tunnel: w348 -> [_ w367]
                  frame False {
                  }
                  frame True {
                    n153 = Build Array (concatenate)(w368, w367) -> (w366:string[])
                    n154 = call "[FGV] Template.vi"("Image Name Array"=w366, "Image Array"=w366, "Command"=enum16{"Initialize", "Save", "Read"}."Save") -> ()  [unwired: 6 in, 3 out]
                  }
                }
                n155 = invoke on="Vision_Image" class="ImageControl" method="Clear ROI"(error in=w337) -> ()  [unwired: 2 in, 3 out]
                n156 = Unbundle By Name(w355) -> ("code"=w360:i32)
                n157 = call "IMAQ Create"("Image Name"=w348) -> ("New Image"=w353:T3, "error out"=w354:errorcluster)  [unwired: 4 in]
                n158 = call "IMAQ Copy"("error in (no error)"=w354, "Image Dst"=w353, "Image Src"=w346) -> ("Image Dst Out"=w352:T3)  [unwired: 3 in, 1 out]
                n159 = Equal?(x=w360, y=-1074395252) -> (x = y?=w358:bool)
                n160 = local read "Curve Extraction"() -> (w335:T5)
                n161 = case shown="False" w358 {
                  tunnel: w361 -> [w374 _]
                  tunnel: w346 -> [w373 w377]
                  tunnel: [w370 w377] -> _
                  tunnel: w352 -> [w370 _]
                  tunnel: [w370 T3 refnum ("Image Dst Out")] -> w332
                  tunnel: w355 -> [w371 w375]
                  tunnel: [w371 w375] -> w334
                  frame False {
                    n162 = property on="Done" class="Bool"("DisabledEnum"=T16."Enabled" ("Disabled")) -> ()  [unwired: 2 in, 2 out]
                    n163 = call-poly "IMAQ Write File 2"("File Path"=w374, "Image"=w373) -> ()  [unwired: 8 in, 2 out]
                  }
                  frame True {
                    n164 = One Button Dialog(message="Invalid learn setup data.\nplease Reset Set", button name ("OK")="OK") -> ()  [unwired: 1 out]
                  }
                }
                n165 = call "Draw Curve.vi"("error in (no error)"=w334, "Curve Extraction"=w335, "Refnum in"=w332) -> ("error out"=w333:errorcluster, "Refnum out"=w331:T3)  [unwired: 7 in]
                "Template Image" <- w331
                n166 = call <vilib>:"Unset Busy.vi"("error in (no error)"=w333) -> ()  [unwired: 10 in, 1 out]
              }
            }
          }
        }
      }
      frame "SetROI" {
        n167 = property on="Vision_Image" class="ImageControl"() -> ("ROI"=w383:T1)  [unwired: 2 in, 2 out]
        n168 = Unbundle By Name(w383) -> ("Global Rectangle"=w385:i32[])
        n169 = Array Size(array=w385) -> (size(s)=w386:i32)
        n170 = Not Equal To 0?(x=w386) -> (x != 0?=w384:bool)
        n171 = case shown="True" w384 {
          tunnel: w383 -> [_ w388]
          frame False {
            n172 = One Button Dialog(message="Please Select An Area As ROI") -> ()  [unwired: 1 in, 1 out]
          }
          frame True {
            n173 = disable-structure shown="Enabled" {
              disable-tunnel: w388 -> [w389 _]
              frame Enabled {
                n174 = local write "ROI"(w389) -> ()
              }
              frame Disabled {
              }
            }
          }
        }
      }
      frame "ClearOverlay" {
        n175 = local read "Vision_Image"() -> (w394:T3)
        n176 = call "IMAQ Clear Overlay"("Image"=w394) -> ("Image Out"=w393:T3)  [unwired: 9 in, 1 out]
        n177 = local write "Vision_Image"(w393) -> ()
      }
      frame "Load Template" {
        # "這個不需要改，因為這是開放給使用者自己去選的"
        # "後面不需要去做Learn Pattern的動作，因為讀進的Pattern都是已經Learn過"
        n178 = Build Path(base path=w403, name or relative path="\\Data") -> (appended path=w402:path)
        n179 = call "File Dialog"("start path"=w402) -> ("selected path"=w401:path, "cancelled"=w400:bool, "error out"=w399:errorcluster)  [unwired: 11 in, 1 out]
        n180 = call <vilib>:"Clear Errors.vi"("error in (no error)"=w399) -> ()  [unwired: 5 in, 2 out]
        n181 = case shown="False" w400 {
          tunnel: w404 -> [w410 w411]
          tunnel: [w409 w411] -> w396
          tunnel: w401 -> [w408 _]
          frame False {
            n182 = call "PatternMatch_ReadTemplate.vi"("template path"=w408, "Template"=w410) -> ("Template Out"=w409:T3)  [unwired: 8 in, 1 out]
          }
          frame True {
          }
        }
        n183 = local write "Template Image"(w396) -> ()
        n184 = call "IMAQ ImageToArray"("Image"=w396) -> ("Image Pixels (U8)"=w397:u8[][])  [unwired: 3 in, 4 out]
        n185 = Empty Array?(array=w397) -> (empty?=w395:bool)
        n186 = case shown="False" w395 {
          frame False {
            n187 = property on="Done" class="Bool"("DisabledEnum"=T16."Enabled" ("Disabled")) -> ()  [unwired: 2 in, 2 out]
          }
          frame True {
          }
        }
      }
      frame "Offset" {
        n188 = local read "ProjectName"() -> (w422:string)
        n189 = Build Path(base path=w425, name or relative path=w422) -> (appended path=w423:path)
        n190 = Build Path(base path=w423, name or relative path=w424) -> (appended path=w428:path)
        n191 = local read "Curve Extraction"() -> (w412:T5)
        n192 = call <vilib>:"Set Busy.vi"() -> ("error out"=w416:errorcluster)  [unwired: 10 in, 1 out]
        n193 = call "IMAQ Setup Learn Geometric Pattern 2"("error in (no error)"=w416, "Curve Parameters"=w412) -> ("error out"=w421:errorcluster, "Learn Geometric Pattern 2 Setup Data"=w420:string)
        n194 = Bundle("X Position Offset"="X Position Offset", "Y Position Offset"="Y Position Offset") -> (w413:T21)  [unwired: 1 in]
        n195 = call "IMAQ Learn Geometric Pattern 3"("Template Image"=w419, "Origin Offset"=w413, "Learn Geometric Pattern 2 Setup Data"=w420, "error in (no error)"=w421) -> ("Template Image Out"=w418:T3, "error out"=w417:errorcluster)  [unwired: 10 in]
        n196 = Unbundle By Name(w417) -> ("code"=w430:i32)
        n197 = Equal?(x=w430, y=-1074395252) -> (x = y?=w431:bool)
        n198 = case shown="False" w431 {
          tunnel: w428 -> [w435 _]
          tunnel: w418 -> [w434 w437]
          tunnel: [w434 w437] -> w426
          tunnel: w417 -> [w432 w436]
          tunnel: [w432 w436] -> w427
          frame False {
            n199 = call-poly "IMAQ Write File 2"("File Path"=w435, "Image"=w434) -> ()  [unwired: 8 in, 2 out]
            n200 = property on="Done" class="Bool"("DisabledEnum"=T16."Enabled" ("Disabled")) -> ()  [unwired: 2 in, 2 out]
          }
          frame True {
            n201 = One Button Dialog(message="Invalid learn setup data.\nplease Reset Set", button name ("OK")="OK") -> ()  [unwired: 1 out]
          }
        }
        n202 = call <vilib>:"Unset Busy.vi"("error in (no error)"=w427) -> ()  [unwired: 10 in, 1 out]
      }
      frame "Draw Curve" {
        n203 = call "IMAQ Clear Overlay"("Image"=w447) -> ("Image Out"=w443:T3)  [unwired: 9 in, 1 out]
        n204 = case shown="True" "Show Curve" {
          tunnel: w443 -> [w448 w451]
          tunnel: "Curve Extraction" -> [_ w450]
          tunnel: [w448 w449] -> w441
          frame False {
          }
          frame True {
            n205 = call "Draw Curve.vi"("Curve Extraction"=w450, "Refnum in"=w451) -> ("Refnum out"=w449:T3)  [unwired: 8 in, 1 out]
          }
        }
        n206 = local write "Vision_Image"(w441) -> ()
      }
    }
    n207 = call <vilib>:"Clear Errors.vi"("error in (no error)"=w50) -> ("error out"=w51:errorcluster)  [unwired: 5 in, 1 out]
  }
  "error out" <- w2
  "IMAQ Curve Parameters.ctlCancel?" <- w37
  n208 = while {
    tunnel: w26 -> [w455]
    tunnel: w11 -> [w454]
    tunnel: w17 -> [w453]
    tunnel: [w452] -> w13
    stop <- w456 stop-if-true
    n209 = event shown="[5] \"Run Algorithm\": Value Change" {
      selector: w453 -> [_ _ _ _ _ _ _ _ _ _ _ _]
      dyn-events: [_ _ _ _ _ _ _ _ _ _ _ _] -> w452
      timeout: _ -> [_ _ _ _ _ _ _ _ _ _ _ _]
      tunnel: [_ TRUE TRUE TRUE _ _ _ _ _ _ _ _] -> w456
      tunnel: w455 -> [_ w459 w463 w467 w470 w476 w481 w493 w495 _ w504 w507]
      tunnel: w454 -> [_ w458 w462 w466 _ w475 w480 w492 w494 _ w503 w506]
      event Timeout {
        n210 = event-data() -> ()  [unwired: 1 in, 2 out]
      }
      event "Done": Value Change {
        n211 = event-data() -> ()  [unwired: 1 in, 6 out]
        n212 = Enqueue Element(queue=w459, element=Pattern_Match_UI_Command."Done", error in (no error)=w458) -> ()  [unwired: 1 in, 3 out]
      }
      event "Cancel": Value Change {
        n213 = event-data() -> ()  [unwired: 1 in, 6 out]
        n214 = Enqueue Element(queue=w463, element=Pattern_Match_UI_Command."Cancel", error in (no error)=w462) -> ()  [unwired: 1 in, 3 out]
      }
      event User Event {
        n215 = event-data() -> ()  [unwired: 1 in, 1 out]
        n216 = Enqueue Element(queue=w467, element=Pattern_Match_UI_Command."Cancel", error in (no error)=w466) -> ()  [unwired: 1 in, 3 out]
      }
      event "Curve Extraction", "Show Curve": Value Change {
        n217 = event-data() -> ()  [unwired: 1 in, 6 out]
        n218 = Enqueue Element(queue=w470, element=Pattern_Match_UI_Command."Draw Curve") -> ()  [unwired: 2 in, 3 out]
      }
      event "Run Algorithm": Value Change {
        n219 = event-data() -> ()  [unwired: 1 in, 6 out]
        n220 = Enqueue Element(queue=w476, element=Pattern_Match_UI_Command."RunAlgorithm", error in (no error)=w475) -> (queue out=w472:refnum<queue>, error out=w473:errorcluster)  [unwired: 1 in, 1 out]
        n221 = Enqueue Element(queue=w472, element=Pattern_Match_UI_Command."Draw Overlay", error in (no error)=w473) -> ()  [unwired: 1 in, 3 out]
      }
      event "SetTemplate": Value Change {
        n222 = event-data() -> ()  [unwired: 1 in, 6 out]
        n223 = Enqueue Element(queue=w481, element=Pattern_Match_UI_Command."SetTemplate", error in (no error)=w480) -> (queue out=w478:refnum<queue>, error out=w477:errorcluster)  [unwired: 1 in, 1 out]
        n224 = disable-structure shown="Enabled" {
          disable-tunnel: w478 -> [w484 _]
          disable-tunnel: w477 -> [w483 _]
          frame Disabled {
            n225 = Enqueue Element(queue=w484, element=T22."RunAlgorithm", error in (no error)=w483) -> ()  [unwired: 1 in, 3 out]
          }
          frame Enabled {
          }
        }
      }
      event "SetROI": Value Change {
        n226 = event-data() -> ()  [unwired: 1 in, 6 out]
        n227 = Enqueue Element(queue=w493, element=Pattern_Match_UI_Command."SetROI", error in (no error)=w492) -> (queue out=w490:refnum<queue>, error out=w489:errorcluster)  [unwired: 1 in, 1 out]
        n228 = Enqueue Element(queue=w490, element=Pattern_Match_UI_Command."RunAlgorithm", error in (no error)=w489) -> (queue out=w486:refnum<queue>, error out=w487:errorcluster)  [unwired: 1 in, 1 out]
        n229 = Enqueue Element(queue=w486, element=Pattern_Match_UI_Command."Draw Overlay", error in (no error)=w487) -> ()  [unwired: 1 in, 3 out]
      }
      event "Vision_Image": Mouse Up {
        w496 = i32[] [2] items=["No Event"=0, "Click Event"=1, "Draw Event"=2, "Size Event"=4, "Scroll Event"=5, "Double Click Event"=8] ("Which Events")
        n230 = event-data() -> ()  [unwired: 1 in, 8 out]
        n231 = invoke on="Vision_Image" class="ImageControl" method="Get Last Event"("Which Events"=w496) -> ("Type"=w497:i32)  [unwired: 7 in, 7 out]
        n232 = Not Equal To 0?(x=w497) -> (x != 0?=w498:bool)
        n233 = case shown="False" w498 {
          tunnel: w495 -> [_ w501]
          tunnel: w494 -> [_ w500]
          frame False {
          }
          frame True {
            n234 = Enqueue Element(queue=w501, element=Pattern_Match_UI_Command."ClearOverlay", error in (no error)=w500) -> ()  [unwired: 1 in, 3 out]
          }
        }
      }
      event "Vision_Image": Mouse Down {
        n235 = event-data() -> ()  [unwired: 1 in, 8 out]
      }
      event Menu Selection (User) {
        n236 = event-data() -> ()  [unwired: 1 in, 8 out]
        n237 = Enqueue Element(queue=w504, element=Pattern_Match_UI_Command."Load Template", error in (no error)=w503) -> ()  [unwired: 1 in, 3 out]
      }
      event "X Position Offset", "Y Position Offset": Value Change {
        n238 = event-data() -> ()  [unwired: 1 in, 6 out]
        n239 = Enqueue Element(queue=w507, element=Pattern_Match_UI_Command."Offset", error in (no error)=w506) -> ()  [unwired: 1 in, 3 out]
      }
    }
  }
  n240 = Unregister For Events(event registration refnum=w13) -> ()  [unwired: 1 in, 1 out]
  n241 = disable-structure shown="Disabled" {
    disable-tunnel: w38 -> [w508 _]
    frame Disabled {
      n242 = call "IMAQ Dispose"("Image"=w508) -> ("error out"=w509:errorcluster)  [unwired: 5 in]
      n243 = call <vilib>:"General Error Handler.vi"("error in (no error)"=w509) -> ()  [unwired: 2 in, 13 out]
    }
    frame Enabled {
    }
  }
  n244 = Destroy User Event(user event=w14) -> (error out=w10:errorcluster)  [unwired: 1 in]
  n245 = call "IMAQ Dispose"("Image"="Pattern Matching Image" ("Image Name"), "error in (no error)"=w10) -> ("error out"=w8:errorcluster)  [unwired: 4 in]
  n246 = Flush Queue(queue=w25) -> (queue out=w28:refnum<queue>, error out=w27:errorcluster)  [unwired: 1 in, 1 out]
  n247 = call "IMAQ Dispose"("Image"="Pattern Matching Template" ("Image Name"), "error in (no error)"=w8) -> ()  [unwired: 4 in, 1 out]
  n248 = Release Queue(queue=w28, error in (no error)=w27) -> ()  [unwired: 1 in, 3 out]
